vi "command to matlab.vi"(1 "Command":string) -> (0 "error out":errorcluster)   [LabVIEW 2013]
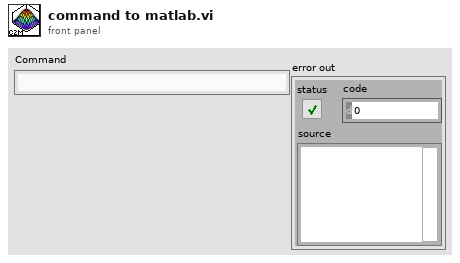
[diagram p1: front panel]
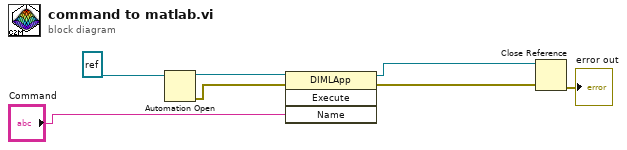
[diagram p0: block diagram]
diagram:
  n1 = Automation Open(Automation Refnum=refnum<k7> refnum ("MLApp.DIMLApp")) -> (Automation Refnum=w5:refnum<k7>, error out=w4:errorcluster)  [unwired: 3 in]
  n2 = invoke class="DIMLApp" method="Execute"(reference=w5, error in=w4, "Name"="Command") -> (reference out=w3:refnum<k7>, error out=w2:errorcluster)  [unwired: 1 in, 2 out]
  n3 = Close Reference(reference=w3, error in (no error)=w2) -> (error out=→"error out":errorcluster)
